vi "Main.vi"(8 "error in":errorcluster, 11 "First Level Worker in":refnum<class "First Level Worker.lvclass">) -> (0 "error out":errorcluster, 3 "First Level Worker out":refnum<class "First Level Worker.lvclass">)   [LabVIEW 2017, in "Method 3.lvlib" / "First Level Worker.lvclass"]
doc: "The <b>Queued Message Handler</b> of the Worker that owns this VI."
uses:
  First Level Worker.lvclass
  First Level Worker.lvclass/First Level Worker.ctl
  Initialization Data.ctl
  Response Cases.ctl
  Second Level Worker/Second Level Worker.lvclass
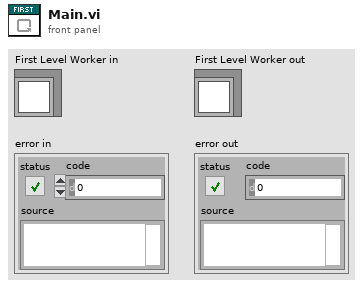
[diagram p1: front panel]
types:
  T1 = typedef "Method 3.lvlib/First Level Worker.lvclass/Initialization Data.ctl" = cluster{"Response Cases":T2}
  T2 = typedef "Method 3.lvlib/First Level Worker.lvclass/Response Cases.ctl" = cluster{"Placeholder - Can be deleted":string}
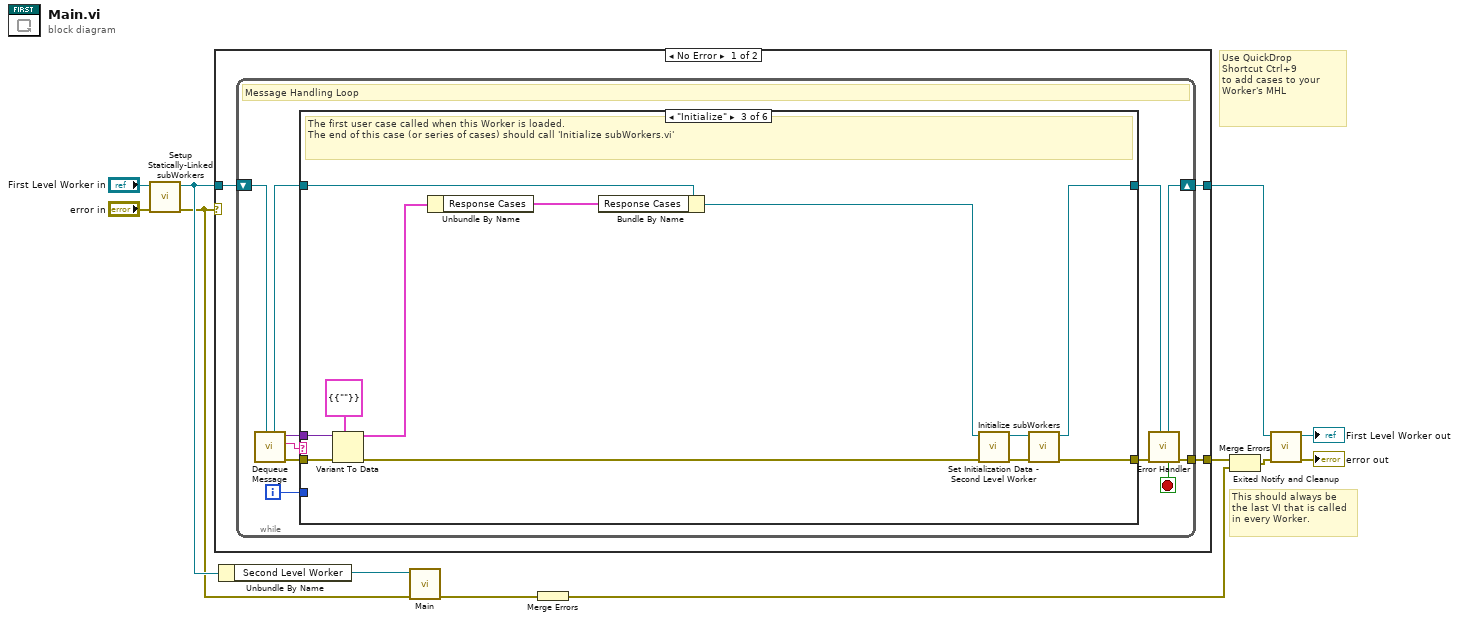
[diagram p0: block diagram]
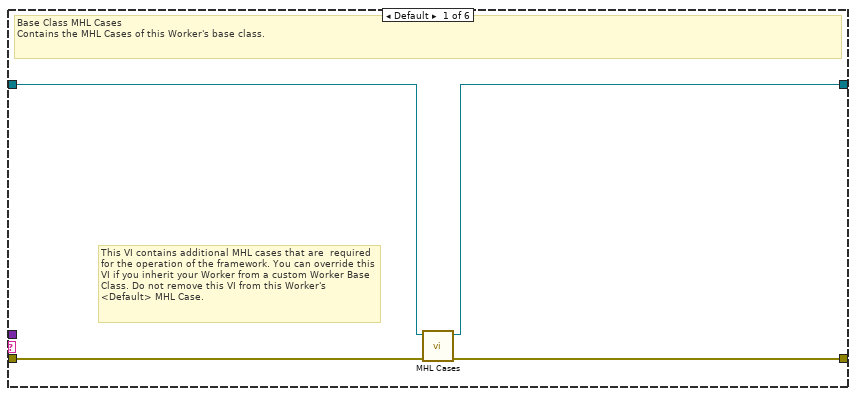
[diagram p2: hidden frame]
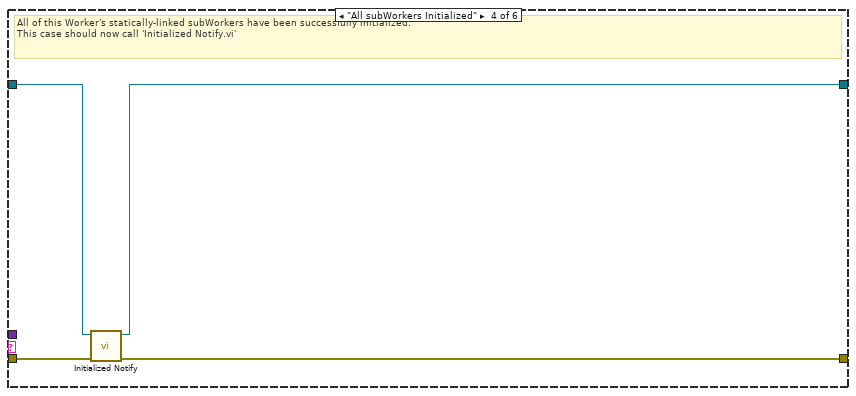
[diagram p4: hidden frame]
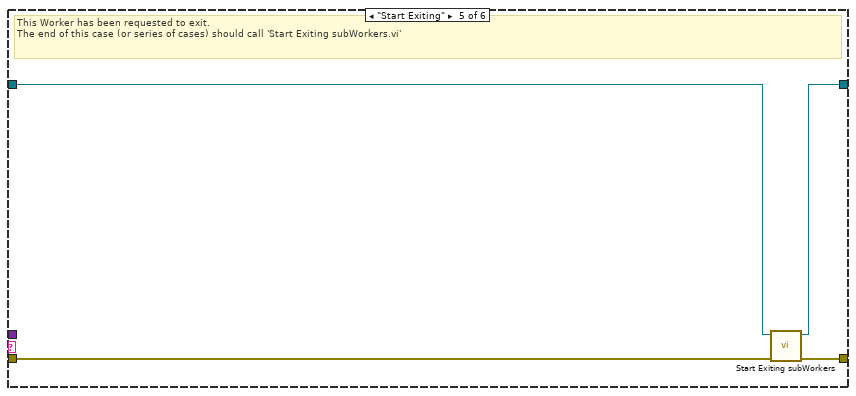
[diagram p5: hidden frame]
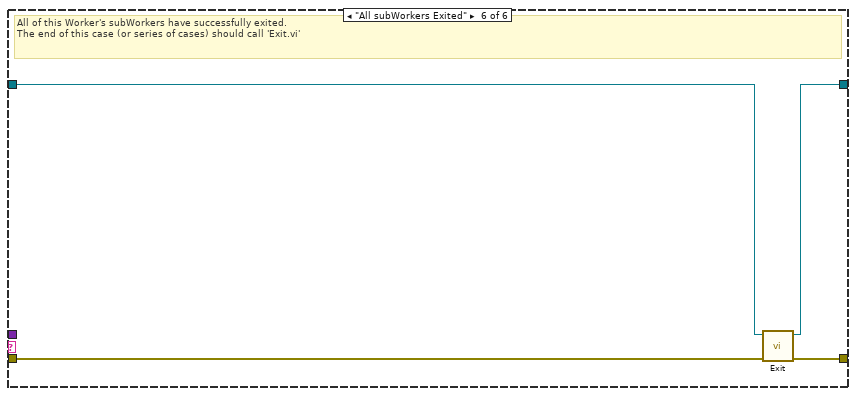
[diagram p6: hidden frame]
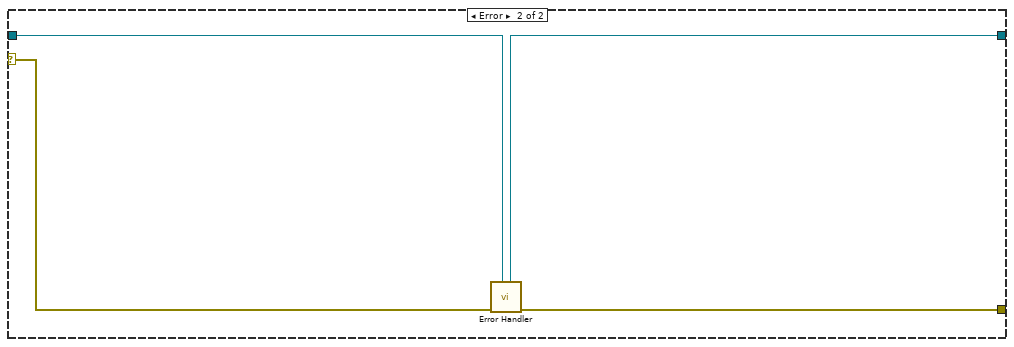
[diagram p7: hidden frame]
diagram:
  # "Use QuickDrop\nShortcut Ctrl+9\nto add cases to your\nWorker's MHL"
  # "This should always be the last VI that is called in every Worker."
  n1 = call "Setup Statically-Linked subWorkers.vi"("error in"="error in", "First Level Worker in"="First Level Worker in") -> ("error out"=w3:errorcluster, "First Level Worker out"=w4:refnum<class "First Level Worker.lvclass">)  [unwired: 8 in]
  n2 = case shown="No Error" w3 {
    tunnel: w4 -> [w15 w58]
    tunnel: [w13 w59] -> w10
    tunnel: [w14 w57] -> w11
    selector: w3 -> [_ w60]
    frame No Error {
      n3 = while {
        shift-right: [w24] -> w14
        shift-left: w15 -> [w26]
        tunnel: [w25] -> w13
        i -> [w16]
        stop <- w17 stop-if-true
        # "Message Handling Loop"
        n4 = call-dynamic "Dequeue Message.vi"("Worker"=w26) -> ("error out"=w23:errorcluster, "Case out"=w18:string, "Data out"=w19:variant, "Worker out"=w21:refnum<class "First Level Worker.lvclass">)  [unwired: 6 in, 1 out]
        n5 = case "Worker MHL Case Structure (DO NOT CHANGE LABEL NAME)" shown="\"Initialize\"" w18 {
          tunnel: w23 -> [w30 w31 w42 w46 w49 w56]
          tunnel: [w29 w31 w44 w45 w52 w55] -> w22
          tunnel: w21 -> [w28 w32 w41 w48 w50 w54]
          tunnel: [w27 w32 w43 w47 w51 w53] -> w20
          tunnel: w19 -> [_ _ w39 _ _ _]
          tunnel: w16 -> [_ _ _ _ _ _]
          frame Default {
            # "This VI contains additional MHL cases that are  required for the operation of the framework. You can override this VI if you inherit your Worker from a custom Worker Base Class. Do not remove this VI from this Worker's <Default> MHL Case."
            # "Base Class MHL Cases\nContains the MHL Cases of this Worker's base class."
            n6 = call-dynamic "MHL Cases.vi"("error in"=w30, "Worker Base Class in"=w28) -> ("error out"=w29:errorcluster, "Worker Base Class out"=w27:refnum<class "First Level Worker.lvclass">)  [unwired: 8 in]
          }
          frame "------------ FRAMEWORK CASES -----------" {
            # "Start of Workers Framework Cases"
          }
          frame "Initialize" {
            # "The first user case called when this Worker is loaded.\nThe end of this case (or series of cases) should call 'Initialize subWorkers.vi'"
            n7 = Variant To Data(error in=w42, type=T1 {"Response Cases"={"Placeholder - Can be deleted"=""}} ("Initialization Data"), Variant=w39) -> (data=w38:T1, error out=w40:errorcluster)
            n8 = Unbundle By Name(w38) -> ("Response Cases"=w37:T2)
            n9 = Bundle By Name(cluster=w41, "Response Cases"=w37) -> (w33:refnum<class "First Level Worker.lvclass">)
            n10 = call "Set Initialization Data - Second Level Worker.vi"("error in"=w40, "First Level Worker in"=w33) -> ("error out"=w35:errorcluster, "First Level Worker out"=w34:refnum<class "First Level Worker.lvclass">)  [unwired: 8 in]
            n11 = call-dynamic "Initialize subWorkers.vi"("error in"=w35, "Worker"=w34) -> ("error out"=w44:errorcluster, "dup Worker out"=w43:refnum<class "First Level Worker.lvclass">)  [unwired: 8 in]
          }
          frame "All subWorkers Initialized" {
            # "All of this Worker's statically-linked subWorkers have been successfully initialized.\nThis case should now call 'Initialized Notify.vi'"
            n12 = call-dynamic "Initialized Notify.vi"("error in"=w46, "Worker"=w48) -> ("error out"=w45:errorcluster, "dup Worker out"=w47:refnum<class "First Level Worker.lvclass">)  [unwired: 8 in]
          }
          frame "Start Exiting" {
            # "This Worker has been requested to exit. \nThe end of this case (or series of cases) should call 'Start Exiting subWorkers.vi'"
            n13 = call-dynamic "Start Exiting subWorkers.vi"("error_in"=w49, "Worker"=w50) -> ("error out"=w52:errorcluster, "dup Worker out"=w51:refnum<class "First Level Worker.lvclass">)  [unwired: 8 in]
          }
          frame "All subWorkers Exited" {
            # "All of this Worker's subWorkers have successfully exited. \nThe end of this case (or series of cases) should call 'Exit.vi'"
            n14 = call-dynamic "Exit.vi"("error_in"=w56, "Worker"=w54) -> ("error out"=w55:errorcluster, "dup Worker out"=w53:refnum<class "First Level Worker.lvclass">)  [unwired: 8 in]
          }
        }
        n15 = call-dynamic "Error Handler.vi"("Worker"=w20, "error_in"=w22) -> ("error out"=w25:errorcluster, "Stop Loop"=w17:bool, "Worker out"=w24:refnum<class "First Level Worker.lvclass">)  [unwired: 7 in]
      }
    }
    frame Error {
      n16 = call-dynamic "Error Handler.vi"("Worker"=w58, "error_in"=w60) -> ("error out"=w59:errorcluster, "Worker out"=w57:refnum<class "First Level Worker.lvclass">)  [unwired: 7 in, 1 out]
    }
  }
  n17 = Unbundle By Name(w4) -> ("Second Level Worker"=w2:refnum<class "Second Level Worker.lvclass">)
  n18 = call-dynamic "Main.vi"("error in"=w3, "Second Level Worker in"=w2) -> ("error out"=w1:errorcluster)  [unwired: 8 in, 1 out]
  n19 = Merge Errors(w1) -> (w5:errorcluster)
  n20 = Merge Errors(w10, w5) -> (w12:errorcluster)
  n21 = call-dynamic "Exited Notify and Cleanup.vi"("error_in"=w12, "Worker"=w11) -> ("error out"=→"error out":errorcluster, "dup Worker out"=→"First Level Worker out":refnum<class "First Level Worker.lvclass">)  [unwired: 8 in]
